vi "OnOperateClick.vi"(0 "XRef":T16, 1 "Point":T14, 2 "State In":T1) -> (14 "Reply":T12, 15 "Fatal Error Out":T11, 16 "State Out":T1)   [LabVIEW 2020, in "Parallel Diagram Block.xnode"]
uses:
  Parallel Diagram Block.xnode
  <vilib>/XNodeSupport/XNodeInt.ctl
  <vilib>/XNodeSupport/NI_XNodeSupport.lvlib
  <vilib>/XNodeSupport/XNodeXNodeRef.ctl
  <vilib>/XNodeSupport/XNodePoint.ctl
  <vilib>/XNodeSupport/XNodeString.ctl
  <vilib>/XNodeSupport/XNodeStringArray.ctl
  <vilib>/XNodeSupport/XNodeErrorCluster.ctl
  State.ctl
  Parallel Block/Value Type.ctl
  Parallel Block/Parallel Block.lvlib
  Parallel Block/Type Descriptor.ctl
  <vilib>/picture/picture.llb/imagedata.ctl
  Parallel Block/Direction.ctl
  Parallel Block/Terminal Mode.ctl
  Parallel Block/Terminal Type.ctl
  Parallel Block/Type Mode.ctl
  Parallel Block/Value Mode.ctl
  Parallel Block/Manager Node.ctl
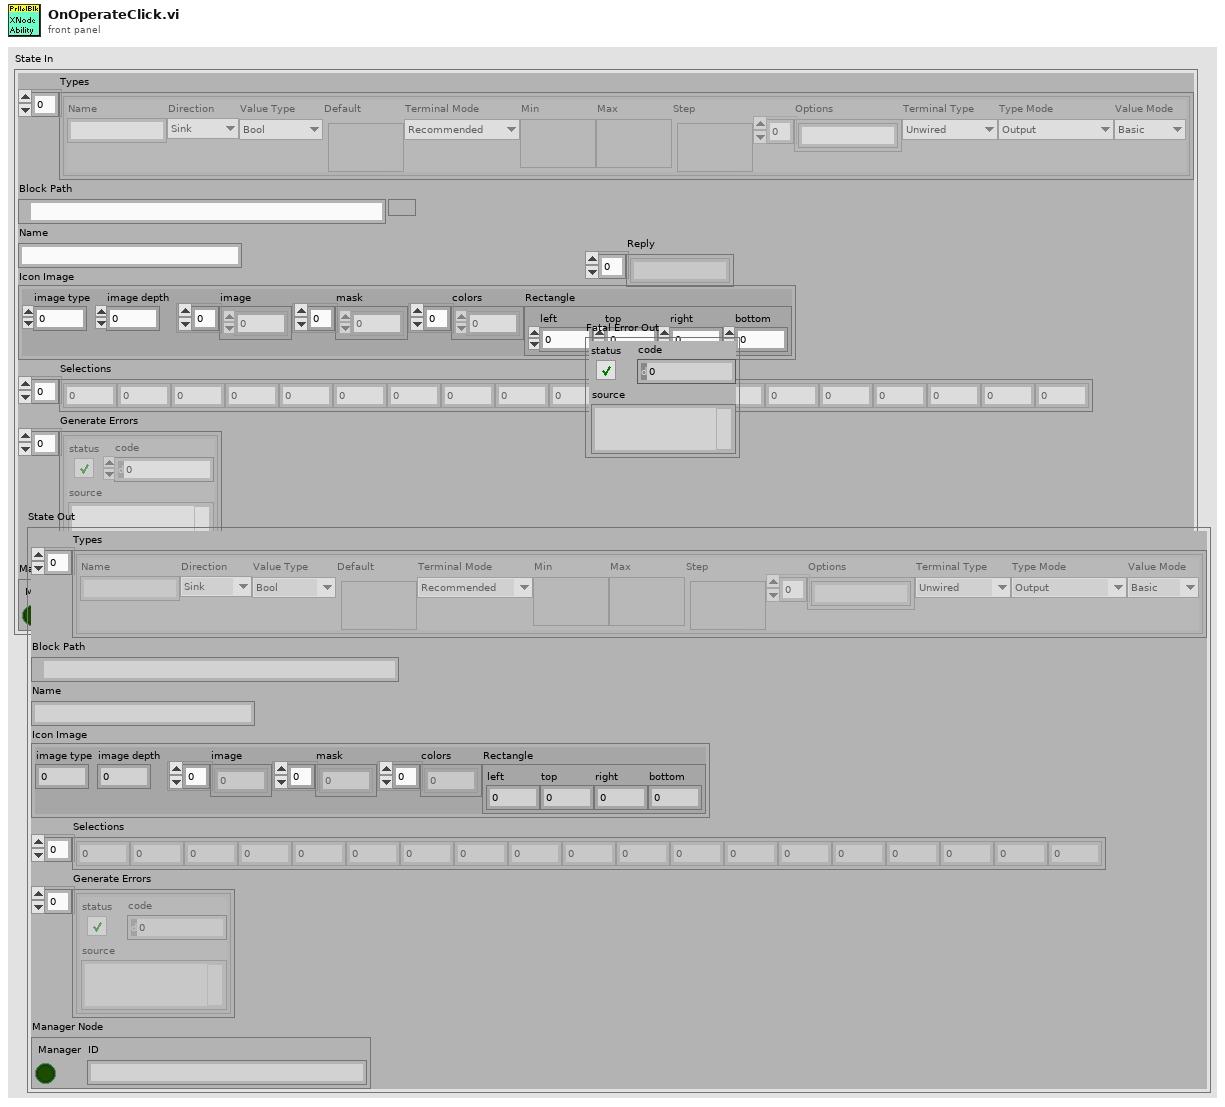
[diagram p1: front panel]
types:
  T1 = typedef "Parallel Diagram Block.xnode/State.ctl" = cluster{"Types":T2[], "Block Path":path, "Name":string, "Icon Image":T9, "Selections":i32[], "Generate Errors":errorcluster[], "Manager Node":T10}
  T2 = typedef "Parallel Block.lvlib/Type Descriptor.ctl" = cluster{"Name":string, "Direction":T3, "Value Type":T4, "Default":variant, "Terminal Mode":T5, "Min":variant, "Max":variant, "Step":variant, "Options":string[], "Terminal Type":T6, "Type Mode":T7, "Value Mode":T8}
  T3 = typedef "Parallel Block.lvlib/Direction.ctl" = enum16{"Sink", "Source"}
  T4 = typedef "Parallel Block.lvlib/Value Type.ctl" = enum16{"Unknown", "Bool", "U8", "U16", "U32", "U64", "I8", "I16", "I32", "I64", "SGL", "DBL", "CSG", "CDB", "CDBWfm", "String", "DBLWfm"}
  T5 = typedef "Parallel Block.lvlib/Terminal Mode.ctl" = enum16{"Recommended", "Required", "None"}
  T6 = typedef "Parallel Block.lvlib/Terminal Type.ctl" = enum16{"Unwired", "BadType", "Connection", "Value", "Control Ref", "BadRefType"}
  T7 = typedef "Parallel Block.lvlib/Type Mode.ctl" = enum16{"Output", "Single - Strict", "Single - Coerced", "Stream"}
  T8 = typedef "Parallel Block.lvlib/Value Mode.ctl" = enum16{"Basic", "Range", "Select"}
  T9 = typedef "imagedata.ctl" = cluster{"image type":i32, "image depth":i32, "image":u8[], "mask":u8[], "colors":u32[], "Rectangle":cluster{"left":i16, "top":i16, "right":i16, "bottom":i16}}
  T10 = typedef "Parallel Block.lvlib/Manager Node.ctl" = cluster{"Manager":bool, "ID":string}
  T11 = typedef "NI_XNodeSupport.lvlib/XNodeErrorCluster.ctl" = errorcluster
  T12 = typedef "NI_XNodeSupport.lvlib/XNodeStringArray.ctl" = T13[]
  T13 = typedef "NI_XNodeSupport.lvlib/XNodeString.ctl" = string
  T14 = typedef "NI_XNodeSupport.lvlib/XNodePoint.ctl" = cluster{"H":T15, "V":T15}
  T15 = typedef "NI_XNodeSupport.lvlib/XNodeInt.ctl" = i32
  T16 = typedef "NI_XNodeSupport.lvlib/XNodeXNodeRef.ctl" = refnum<vi>
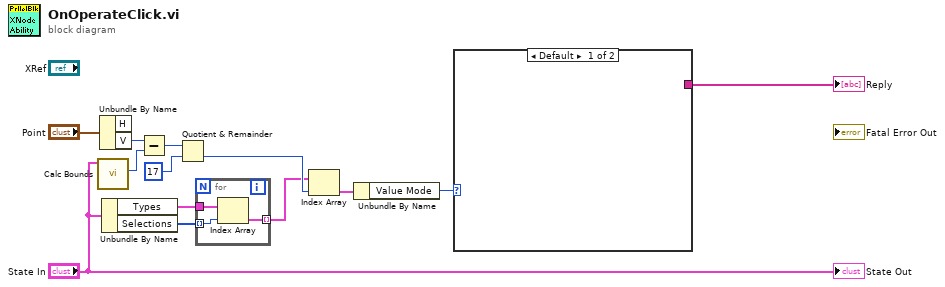
[diagram p0: block diagram]
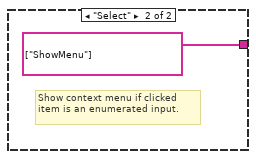
[diagram p2: hidden frame]
diagram:
  n1 = call "Calc Bounds.vi"("State"="State In") -> ("Header"=w10:i32)  [unwired: 4 in, 6 out]
  n2 = Unbundle By Name("Point") -> ("V"=w11:T15)  [unwired: 1 out]
  n3 = Unbundle By Name("State In") -> ("Types"=w3:T2[], "Selections"=w2:i32[])
  n4 = Subtract(x=w11, y=w10) -> (x-y=w9:T15)
  n5 = Quotient & Remainder(x=w9, y=T15 17) -> (floor(x/y)=w7:T15)  [unwired: 1 out]
  n6 = for {
    tunnel: w3 -> [w16]
    tunnel: w2 -> [w15] mode=indexing
    tunnel: [w14] -> w1 mode=indexing
    n7 = Index Array(array=w16, index=w15) -> (element=w14:T2)
  }
  n8 = Index Array(array=w1, index=w7) -> (element=w6:T2)
  n9 = Unbundle By Name(w6) -> ("Value Mode"=w5:T8)
  n10 = case shown="Default" w5 {
    tunnel: [_ string[] ["ShowMenu"]] -> w4
    frame Default {
    }
    frame "Select" {
      # "Show context menu if clicked item is an enumerated input."
    }
  }
  "Reply" <- w4
  "State Out" <- "State In"
